vi "PSU_initialize_2.vi"(7 "safe Mode?":bool, 9 "Current":dbl format="%.2f", 10 "Voltage":dbl format="%.2f", 11 "VISA resource name":refnum<visa-resource-name>="COM5") -> (0 "error out":errorcluster, 3 "VISA resource name out":refnum<visa-resource-name>)   [LabVIEW 2023]
uses:
  <vilib>/Instr/_visa.llb/VISA Configure Serial Port (Instr).vi
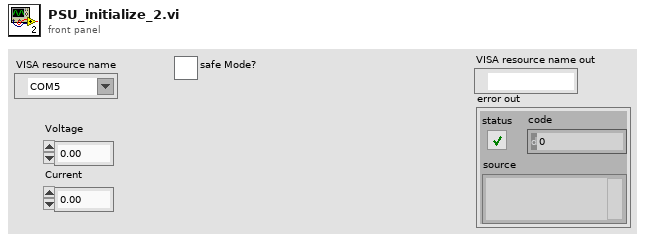
[diagram p1: front panel]
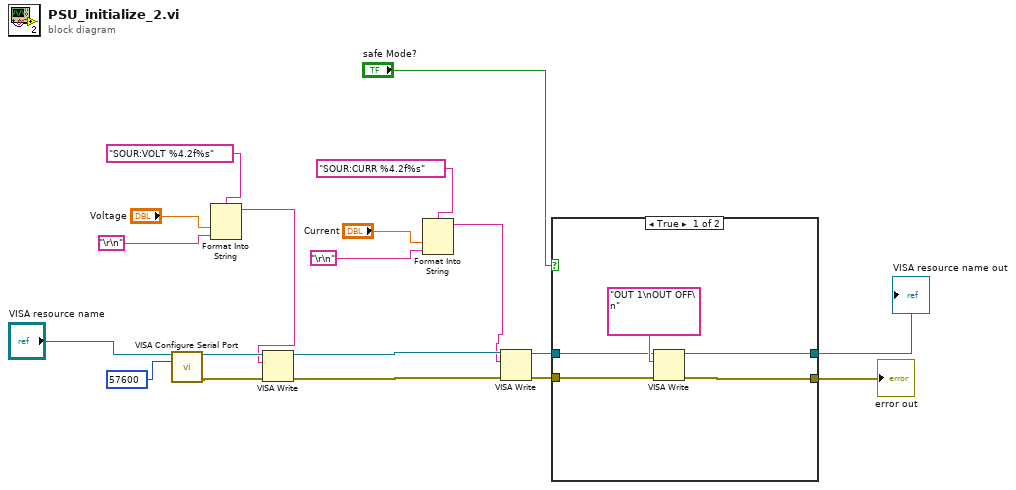
[diagram p0: block diagram]
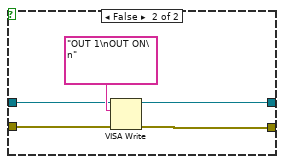
[diagram p2: hidden frame]
diagram:
  n1 = call-poly "VISA Configure Serial Port"("VISA resource name"="VISA resource name", "baud rate (9600)"=u32 57600) -> ("VISA resource name out"=w17:refnum<visa-resource-name>, "error out"=w16:errorcluster)  [unwired: 12 in]
  n2 = Format Into String(format string="SOUR:VOLT %4.2f%s", "Voltage", "\r\n") -> (resulting string=w12:string)  [unwired: 2 in, 1 out]
  n3 = VISA Write(VISA resource name=w17, write buffer=w12, error in (no error)=w16) -> (VISA resource name out=w11:refnum<visa-resource-name>, error out=w10:errorcluster)  [unwired: 1 out]
  n4 = Format Into String(format string="SOUR:CURR %4.2f%s", "Current", "\r\n") -> (resulting string=w6:string)  [unwired: 2 in, 1 out]
  n5 = VISA Write(VISA resource name=w11, write buffer=w6, error in (no error)=w10) -> (VISA resource name out=w5:refnum<visa-resource-name>, error out=w4:errorcluster)  [unwired: 1 out]
  n6 = case shown="True" "safe Mode?" {
    tunnel: w5 -> [w23 w28]
    tunnel: w4 -> [w22 w27]
    tunnel: [w21 w26] -> w3
    tunnel: [w20 w25] -> w2
    frame True {
      n7 = VISA Write(VISA resource name=w23, write buffer="OUT 1\nOUT OFF\n", error in (no error)=w22) -> (VISA resource name out=w21:refnum<visa-resource-name>, error out=w20:errorcluster)  [unwired: 1 out]
    }
    frame False {
      n8 = VISA Write(VISA resource name=w28, write buffer="OUT 1\nOUT ON\n", error in (no error)=w27) -> (VISA resource name out=w26:refnum<visa-resource-name>, error out=w25:errorcluster)  [unwired: 1 out]
    }
  }
  "VISA resource name out" <- w3
  "error out" <- w2
